vi "Reanimate All.vi"(8 "Error In":errorcluster) -> (0 "Error Out":errorcluster)   [LabVIEW 2017, in "Bookmark Manager.lvlib" / "Tests.lvlib"]
uses:
  Tests.lvlib
  Support/Reanimate All Target.vi
  <vilib>/addons/_JKI Toolkits/Caraya/classes/Test/Test.lvclass
  Bookmark Manager.lvlib
  Toolkit/Toolkit.lvlib
  <vilib>/addons/_JKI Toolkits/Caraya/classes/Assert/Assert.lvclass
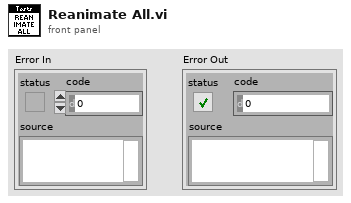
[diagram p1: front panel]
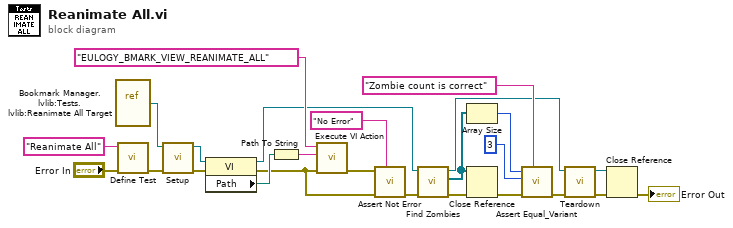
[diagram p0: block diagram]
diagram:
  n1 = vi-ref "Bookmark Manager.lvlib:Tests.lvlib:Reanimate All Target.vi"() -> (w22:refnum<vi>)
  n2 = call <vilib>:"Define Test.vi"("error in (no error)"="Error In", "Label (VI Title)"="Reanimate All") -> ("error out"=w23:errorcluster)  [unwired: 9 in]
  n3 = call "Setup.vi"("Error In"=w23, "VI In"=w22) -> ("Error Out"=w20:errorcluster, "VI Out"=w19:refnum<vi>)  [unwired: 8 in]
  n4 = property class="VI"(reference=w19, error in=w20) -> (reference out=w16:refnum<vi>, error out=w9:errorcluster, "Path"=w18:path)
  n5 = Path To String(path=w18) -> (string=w17:string)
  n6 = call "Execute VI Action.vi"("Error In"=w9, "VI Tree Tag"=w17, "Menu Tag"="EULOGY_BMARK_VIEW_REANIMATE_ALL") -> ("Error Out"=w11:errorcluster)  [unwired: 8 in]
  n7 = call <vilib>:"Assert Not Error.vi"("Label"="No Error", "error in (no error)"=w9, "Not Error?"=w11) -> ("error out"=w10:errorcluster)  [unwired: 8 in]
  n8 = call "Find Zombies.vi"("Error In"=w10, "VI In"=w16) -> ("Error Out"=w13:errorcluster, "Graves"=w1:refnum<vi>[], "VI Out"=w7:refnum<vi>)  [unwired: 7 in]
  n9 = Array Size(array=w1) -> (size(s)=w15:i32)
  n10 = Close Reference(reference=w1, error in (no error)=w13) -> (error out=w2:errorcluster)
  n11 = call <vilib>:"Assert Equal_Variant.vi"("Label"="Zombie count is correct", "error in (no error)"=w2, "Y"=3 ("size(s)"), "X"=w15) -> ("error out"=w8:errorcluster)  [unwired: 7 in]
  n12 = call "Teardown.vi"("Error In"=w8, "VI In"=w7) -> ("Error Out"=w6:errorcluster, "VI Out"=w5:refnum<vi>)  [unwired: 8 in]
  n13 = Close Reference(reference=w5, error in (no error)=w6) -> (error out=→"Error Out":errorcluster)
